vi "986x.Compile.vi"(8 "error in (no error)":errorcluster, 11 "Item Ref in":T2 format="%.0x") -> (0 "error out":errorcluster, 2 "986x Support":T1, 3 "Item Ref out":T2=18446744073709551615 format="%.0x")   [LabVIEW 2015, in "Protection and Counter Addon System Explorer.lvlib"]
uses:
  Protection and Counter Addon System Explorer.lvlib
  <vilib>/NI Veristand/Custom Device API/Custom Device Item Ref.ctl
  Shared/Types/986x.ctl
  <vilib>/NI Veristand/Custom Device API/Get Item Property (String).vi
  Shared/SubVIs/GUID Lookup.vi
  <vilib>/NI Veristand/Custom Device API/Get Item Property (Boolean).vi
  <vilib>/NI VeriStand/Custom Device API/Custom Device API.lvlib
  Shared/Protection and Counter Addon Shared.lvlib
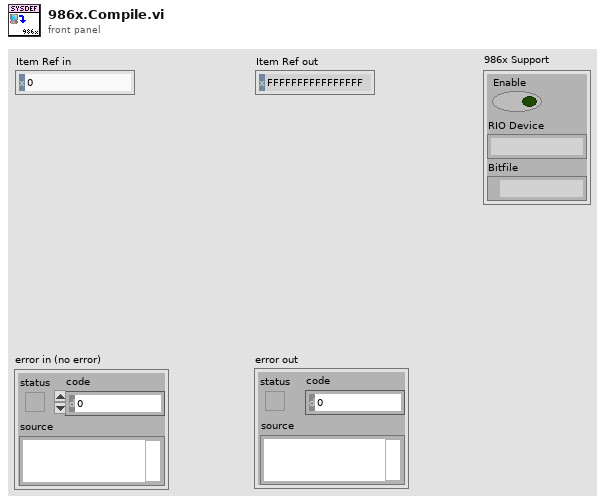
[diagram p1: front panel]
types:
  T1 = typedef "Protection and Counter Addon Shared.lvlib/986x.ctl" = cluster{"Enable":bool, "RIO Device":string, "Bitfile":path}
  T2 = typedef "Custom Device API.lvlib/Custom Device Item Ref.ctl" = u64
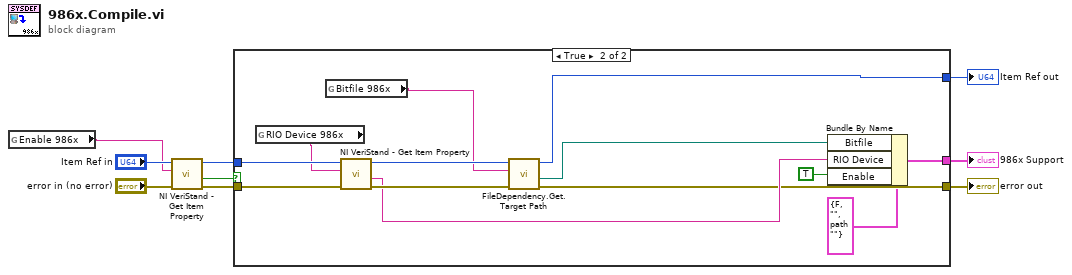
[diagram p0: block diagram]
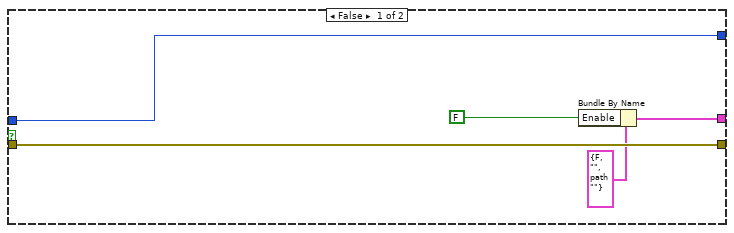
[diagram p2: hidden frame]
diagram:
  n1 = global read "GUID Lookup.vi" "Enable 986x"() -> (w1:string)
  n2 = call-poly <vilib>:"NI VeriStand - Get Item Property.vi"("error in (no error)"="error in (no error)", "Property Name"=w1, "Item Ref in"="Item Ref in") -> ("error out"=w3:errorcluster, "Value"=w4:bool, "Item Ref out"=w9:T2)  [unwired: 5 in, 1 out]
  n3 = case shown="True" w4 {
    tunnel: w9 -> [w13 w25]
    tunnel: w3 -> [w14 w27]
    tunnel: [w14 w21] -> w8
    tunnel: [w13 w19] -> w5
    tunnel: [w12 w23] -> w2
    frame False {
      n4 = Bundle By Name(cluster=T1 {"Enable"=FALSE, "RIO Device"="", "Bitfile"=path ""} ("986x Support"), "Enable"=FALSE) -> (w12:T1)
    }
    frame True {
      n5 = global read "GUID Lookup.vi" "RIO Device 986x"() -> (w16:string)
      n6 = global read "GUID Lookup.vi" "Bitfile 986x"() -> (w15:string)
      n7 = call-poly <vilib>:"NI VeriStand - Get Item Property.vi"("error in (no error)"=w27, "Property Name"=w16, "Item Ref in"=w25) -> ("error out"=w26:errorcluster, "Value"=w24:string, "Item Ref out"=w20:T2)  [unwired: 5 in, 1 out]
      n8 = call "FileDependency.Get.Target Path.vi"("error in (no error)"=w26, "Bitfile 986x"=w15, "Item Ref in"=w20) -> ("error out"=w21:errorcluster, "Target Path"=w18:path, "Item Ref out"=w19:T2)  [unwired: 5 in, 1 out]
      n9 = Bundle By Name(cluster=T1 {"Enable"=FALSE, "RIO Device"="", "Bitfile"=path ""} ("986x Support"), "Bitfile"=w18, "RIO Device"=w24, "Enable"=TRUE) -> (w23:T1)
    }
  }
  "error out" <- w8
  "Item Ref out" <- w5
  "986x Support" <- w2
